vi "sub_qam_demod.vi"(8 "symbol map":cdb[](array[numeric]), 11 "symbol":cdb[](array[numeric])) -> (3 "bitstream":i16[](array[numeric]))   [LabVIEW 2014]
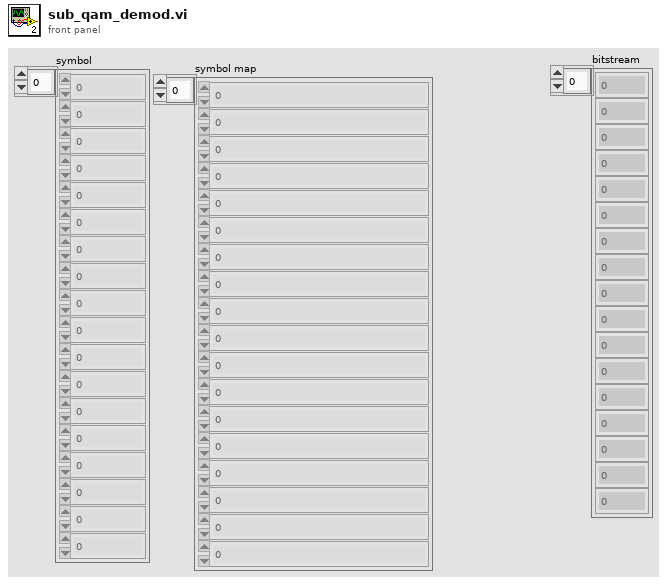
[diagram p1: front panel]
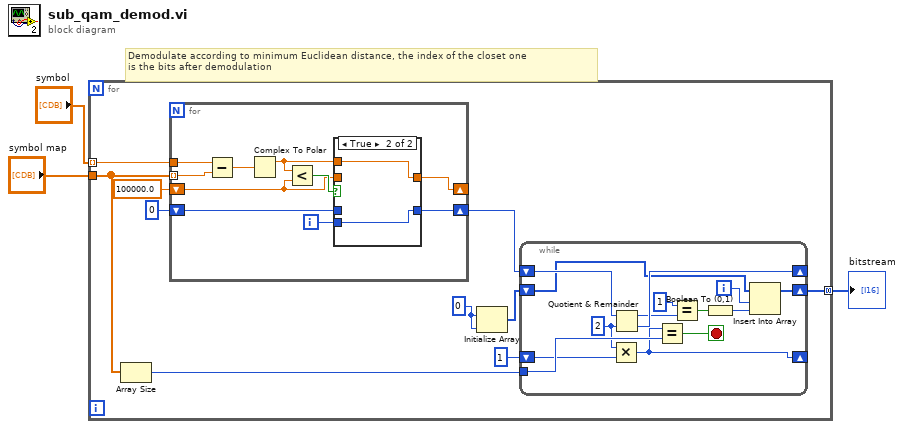
[diagram p0: block diagram]
diagram:
  # "Demodulate according to minimum Euclidean distance, the index of the closet one \nis the bits after demodulation"
  n1 = for {
    tunnel: "symbol" -> [w13] mode=indexing
    tunnel: "symbol map" -> [w5]
    tunnel: [w6] -> w1 mode=concatenating
    w8 = 0
    n2 = Array Size(array=w5) -> (size(s)=w10:i32)
    n3 = for {
      tunnel: w5 -> [w36] mode=indexing
      tunnel: w13 -> [w37]
      shift-right: [w28] -> _
      shift-left: 100000.0 -> [w29]
      shift-right: [w31] -> w4
      shift-left: 0 -> [w33]
      i -> [w34]
      n4 = Subtract(x=w37, y=w36) -> (x-y=w35:cdb)
      n5 = Complex To Polar(r * e^(i*theta)=w35) -> (r=w30:dbl)  [unwired: 1 out]
      n6 = Less?(x=w30, y=w29) -> (x < y?=w32:bool)
      n7 = case shown="True" w32 {
        tunnel: w34 -> [_ w41]
        tunnel: w33 -> [w38 _]
        tunnel: [w38 w41] -> w31
        tunnel: w30 -> [_ w40]
        tunnel: w29 -> [w39 _]
        tunnel: [w39 w40] -> w28
        frame False {
        }
        frame True {
        }
      }
    }
    n8 = Initialize Array(w8, w8) -> (w7:i32[])
    n9 = while {
      tunnel: w10 -> [w27]
      shift-right: [w15] -> _
      shift-left: 1 -> [w26]
      shift-right: [w16] -> w6
      shift-left: w7 -> [w18]
      shift-right: [w22] -> _
      shift-left: w4 -> [w24]
      i -> [w14]
      stop <- w25 stop-if-true
      w23 = 2
      n10 = Multiply(x=w23, y=w26) -> (x*y=w15:i32)
      n11 = Quotient & Remainder(x=w24, y=w23) -> (x-y*floor(x/y)=w20:i32, floor(x/y)=w22:i32)
      n12 = Equal?(x=w15, y=w27) -> (x = y?=w25:bool)
      n13 = Equal?(x=1, y=w20) -> (x = y?=w19:bool)
      n14 = Boolean To (0,1)(Boolean=w19) -> (0, 1=w17:i16)
      n15 = Insert Into Array(array=w18, index=w14, new element=w17) -> (w16:i32[])
    }
  }
  "bitstream" <- w1
